vi "Read Payload.vi"(8 "error in (no error)":errorcluster, 10 "Include Header":bool, 11 "CIFFIFO in":refnum<class "CIF_NIChn_Fifo_U8.lvclass">) -> (0 "error out":errorcluster, 2 "Payload":u8[](array[numeric]))   [LabVIEW 2021, in "CIF_NIChn_Fifo_U8.lvclass"]
uses:
  CIF_NIChn_Fifo_U8.lvclass
  CIF_NIChn_Fifo_U8.lvclass/CIF_NIChn_Fifo_U8.ctl
  ChannelCommon/ChannelCommon.lvlib
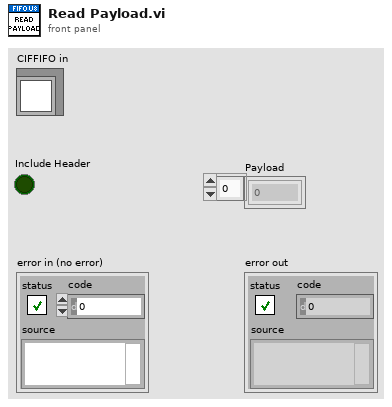
[diagram p1: front panel]
types:
  T1 = typedef "ChannelCommon.lvlib/FIFO Header.ctl" = cluster{"Length":u64, "T0":i64, "T_Out":i64, "T_Tx":i64, "Ctr":u64, "ClockID":u8}
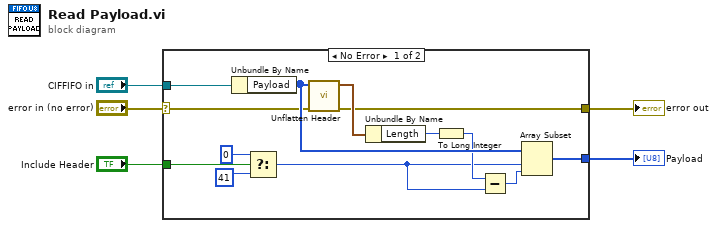
[diagram p0: block diagram]
diagram:
  n1 = case shown="No Error" "error in (no error)" {
    selector: "error in (no error)" -> [w15 w19]
    tunnel: [w14 w19] -> w4
    tunnel: "CIFFIFO in" -> [w16 _]
    tunnel: "Include Header" -> [w10 _]
    tunnel: [w6 _] -> w1
    frame No Error {
      n2 = Unbundle By Name(w16) -> ("Payload"=w18:u8[])
      n3 = Select(t=0, s=w10, f=41 ("index")) -> (s? t:f=w7:i32)
      n4 = call "Unflatten Header.vi"("error in (no error)"=w15, "Flattened Data in"=w18) -> ("error out"=w14:errorcluster, "Header out"=w17:T1)  [unwired: 7 in, 1 out]
      n5 = Unbundle By Name(w17) -> ("Length"=w13:u64)
      n6 = To Long Integer(number=w13) -> (32bit integer=w11:i32)
      n7 = Subtract(x=w11, y=w7) -> (x-y=w12:i32)
      n8 = Array Subset(array=w18, index=w7, length=w12) -> (w6:u8[])
    }
    frame Error {
    }
  }
  "error out" <- w4
  "Payload" <- w1
